vi "设置UI.vi"() -> ()   [LabVIEW 2016]
uses:
  <vilib>/Utility/config.llb/NI_LVConfig.lvlib
panel:
  in  "关闭":bool
  in  "启用":bool
  out "内容":string
  in  "测试":bool
  out "error out":errorcluster caption="错误输出"
  out "body":string caption="体部"
  out "headers":string caption="头部"
  in  "站点":string
  in  "PhoneNumbers":string
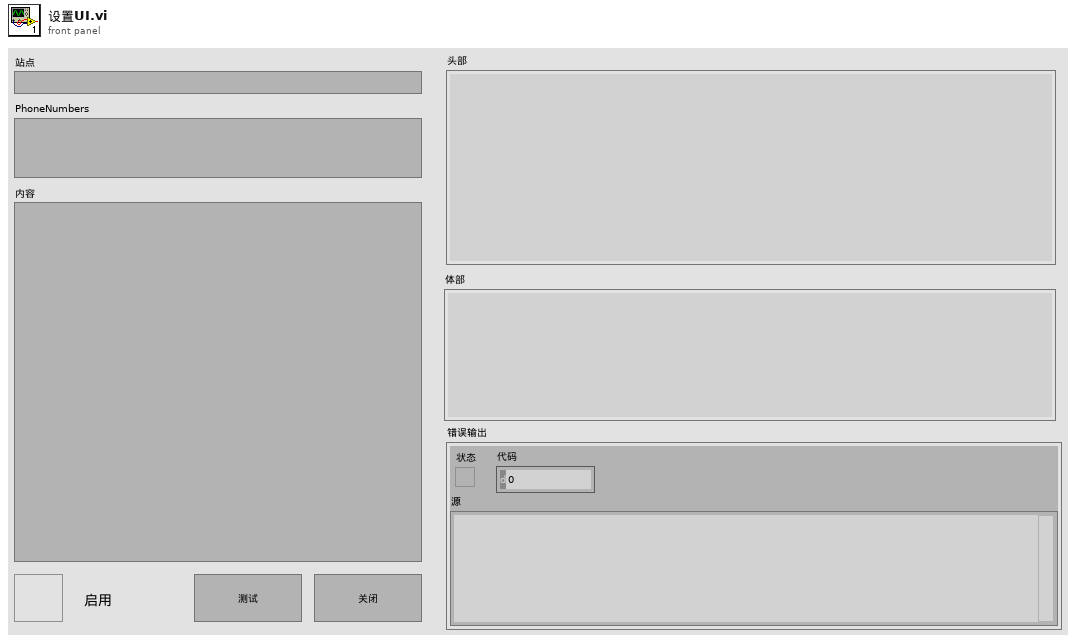
[diagram p1: front panel]
types:
  T1 = typedef "NI_LVConfig.lvlib/Config Data RefNum.ctl" = refnum<k1>
  T2 = enum32{"Invalid", "Standard", "Closed", "Hidden", "Minimized", "Maximized"}
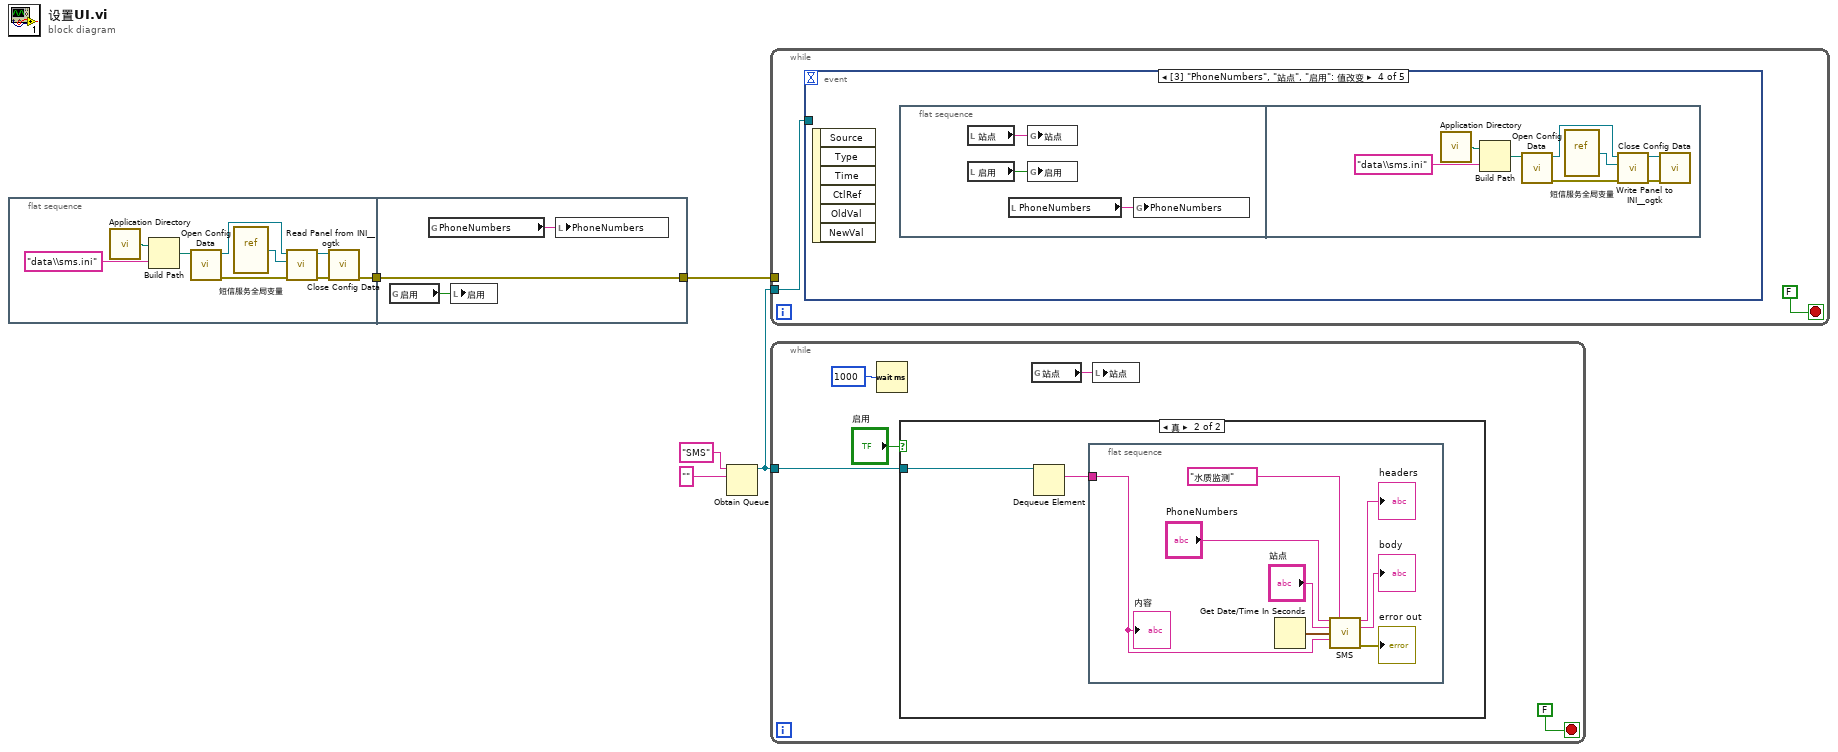
[diagram p0: block diagram]
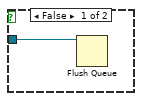
[diagram p2: hidden frame]
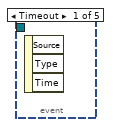
[diagram p3: hidden frame]
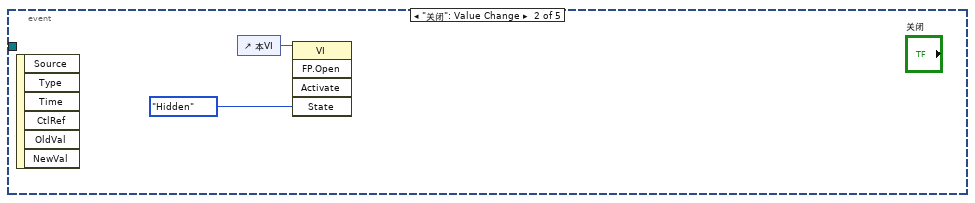
[diagram p4: hidden frame]
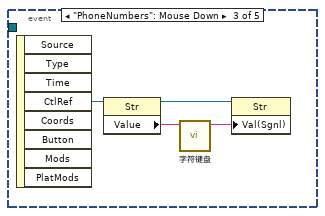
[diagram p5: hidden frame]
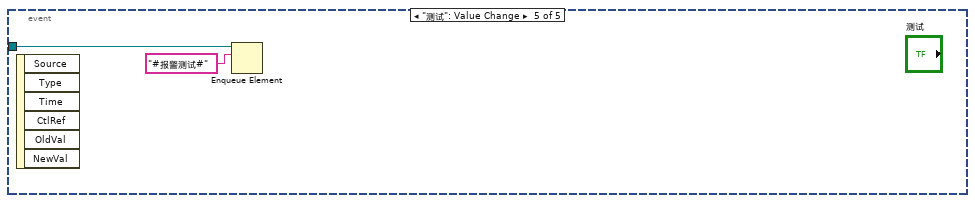
[diagram p6: hidden frame]
diagram:
  n1 = flat-sequence {
    tunnel: [w6] -> w4
    tunnel: [w17] -> w5
    tunnel: w4 -> [w17]
    frame #0 {
      n2 = call <vilib>:"Application Directory.vi"() -> ("Application Directory"=w12:path)
      n3 = Build Path(base path=w12, name or relative path="data\\sms.ini" ("名称或相对路径")) -> (appended path=w13:path)
      n4 = call <vilib>:"Open Config Data.vi"("configuration file path"=w13) -> ("error out"=w8:errorcluster, "refnum"=w7:T1)  [unwired: 8 in, 1 out]
      n5 = vi-ref "短信服务全局变量.vi"() -> (w11:refnum<vi>)
      n6 = call <userlib>:"Read Panel from INI__ogtk.vi"("error in (no error)"=w8, "VI ref"=w11, "refnum"=w7) -> ("error out"=w10:errorcluster, "refnum out"=w9:T1)  [unwired: 7 in]
      n7 = call <vilib>:"Close Config Data.vi"("error in (no error)"=w10, "refnum"=w9) -> ("error out"=w6:errorcluster)  [unwired: 8 in, 1 out]
    }
    frame #1 {
      n8 = global read "短信服务全局变量.vi" "启用"() -> (w15:bool)
      n9 = global read "短信服务全局变量.vi" "PhoneNumbers"() -> (w16:string)
      n10 = local write "启用"(w15) -> ()
      n11 = local write "PhoneNumbers"(w16) -> ()
    }
  }
  n12 = Obtain Queue(name (unnamed)="SMS" ("名称（未命名）"), element data type="" ("名称（未命名）")) -> (queue out=w1:refnum<queue>)  [unwired: 3 in, 2 out]
  n13 = while {
    tunnel: w5 -> [_]
    tunnel: w1 -> [w18]
    stop <- FALSE stop-if-true
    n14 = event shown="[3] \"PhoneNumbers\", \"站点\", \"启用\": 值改变" {
      selector: _ -> [_ _ _ _ _]
      dyn-events: _ -> [_ _ _ _ _]
      timeout: _ -> [_ _ _ _ _]
      tunnel: w18 -> [_ _ _ _ w38]
      event Timeout {
        n15 = event-data() -> ()  [unwired: 1 in, 3 out]
      }
      event "关闭": Value Change {
        n16 = event-data() -> ()  [unwired: 1 in, 6 out]
        n17 = control-ref of="本VI"() -> (w20:refnum<vi>)
        n18 = invoke class="VI" method="FP.Open"(reference=w20, "State"=T2."Hidden" ("状态")) -> ()  [unwired: 3 in, 5 out]
      }
      event "PhoneNumbers": Mouse Down {
        n19 = event-data() -> ("CtlRef"=w25:refnum<vi>)  [unwired: 1 in, 7 out]
        n20 = property class="Str"(reference=w25) -> (reference out=w22:refnum<vi>, "Value"=w24:string)  [unwired: 1 in, 1 out]
        n21 = call "字符键盘.vi"("Old String"=w24) -> ("String"=w23:string)  [unwired: 10 in]
        n22 = property class="Str"(reference=w22, "Val(Sgnl)"=w23) -> ()  [unwired: 1 in, 2 out]
      }
      event "PhoneNumbers", "站点", "启用": Value Change {
        n23 = event-data() -> ()  [unwired: 1 in, 6 out]
        n24 = flat-sequence {
          frame #0 {
            n25 = local read "站点"() -> (w28:string)
            n26 = local read "启用"() -> (w26:bool)
            n27 = local read "PhoneNumbers"() -> (w27:string)
            n28 = global write "短信服务全局变量.vi" "站点"(w28) -> ()
            n29 = global write "短信服务全局变量.vi" "启用"(w26) -> ()
            n30 = global write "短信服务全局变量.vi" "PhoneNumbers"(w27) -> ()
          }
          frame #1 {
            n31 = call <vilib>:"Application Directory.vi"() -> ("Application Directory"=w31:path)
            n32 = Build Path(base path=w31, name or relative path="data\\sms.ini" ("名称或相对路径")) -> (appended path=w30:path)
            n33 = call <vilib>:"Open Config Data.vi"("configuration file path"=w30) -> ("error out"=w35:errorcluster, "refnum"=w36:T1)  [unwired: 8 in, 1 out]
            n34 = vi-ref "短信服务全局变量.vi"() -> (w32:refnum<vi>)
            n35 = call <userlib>:"Write Panel to INI__ogtk.vi"("error in (no error)"=w35, "VI ref"=w32, "refnum"=w36) -> ("error out"=w33:errorcluster, "refnum out"=w34:T1)  [unwired: 7 in]
            n36 = call <vilib>:"Close Config Data.vi"("error in (no error)"=w33, "refnum"=w34) -> ()  [unwired: 8 in, 2 out]
          }
        }
      }
      event "测试": Value Change {
        n37 = event-data() -> ()  [unwired: 1 in, 6 out]
        n38 = Enqueue Element(queue=w38, element="#报警测试#" ("内容")) -> ()  [unwired: 2 in, 3 out]
      }
    }
  }
  n39 = while {
    tunnel: w1 -> [w41]
    stop <- FALSE stop-if-true
    n40 = Wait (ms)(milliseconds to wait=u32 1000 ("等待时间（毫秒）")) -> ()  [unwired: 1 out]
    n41 = case shown="真" "启用" {
      tunnel: w41 -> [w44 w46]
      frame False {
        n42 = Flush Queue(queue=w44) -> ()  [unwired: 1 in, 3 out]
      }
      frame True {
        n43 = Dequeue Element(queue=w46) -> (element=w45:string)  [unwired: 2 in, 3 out]
        n44 = flat-sequence {
          tunnel: w45 -> [w54]
          frame #0 {
            n45 = Get Date/Time In Seconds() -> (seconds since 1Jan1904=w51:timestamp)
            n46 = call "SMS.vi"("PhoneNumbers"="PhoneNumbers", "SignName"="水质监测", "站点"="站点", "时间标识"=w51, "内容"=w54) -> ("headers"=→"headers":string, "body"=→"body":string, "error out"=→"error out":errorcluster)  [unwired: 8 in]
            "内容" <- w54
          }
        }
      }
    }
    n47 = global read "短信服务全局变量.vi" "站点"() -> (w39:string)
    n48 = local write "站点"(w39) -> ()
  }
